vi "GV-progress.vi"() -> (6 "37x37":picture)   [LabVIEW 2020, in "Gviewer.lvclass"]
doc: "Andre Koelewijn, April 2019\n\nThis progress indicator shows loop activity and indicates loop time in msec or seconds.\nExtreme fast loops will increase indicator speed.\nAverage speed loops will show identical indicator speed.\nExtreme slow loops will show by low speed update rate."
uses:
  Gviewer.lvclass
  <vilib>/ptbypt/NI_PtbyPt.lvlib
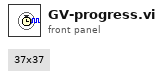
[diagram p1: front panel]
types:
  T1 = cluster{"horizontal":enum16{"left", "center", "right"}, "vertical":enum16{"top", "center", "bottom"}}
  T2 = cluster{"Width":u16, "Style":enum32{"Solid", "Dash", "Dot", "DashDot", "DashDotDot"}}
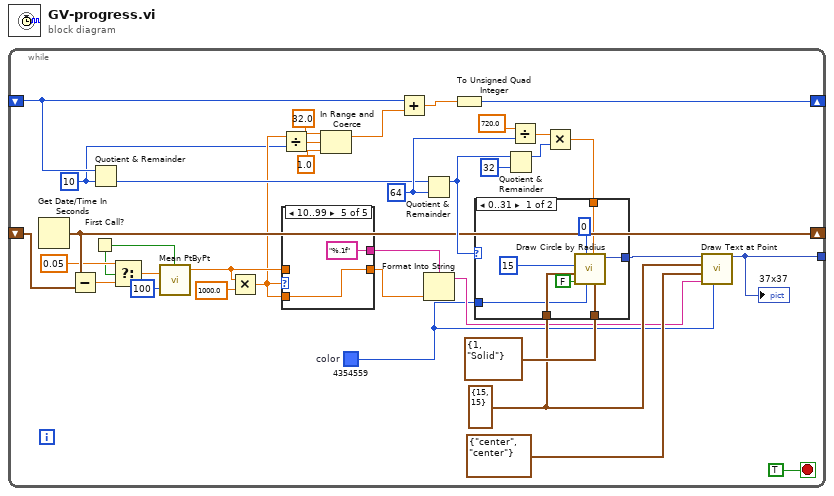
[diagram p0: block diagram]
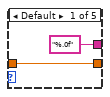
[diagram p2: hidden frame]
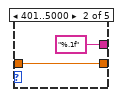
[diagram p3: hidden frame]
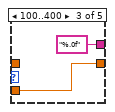
[diagram p4: hidden frame]
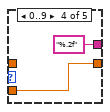
[diagram p5: hidden frame]
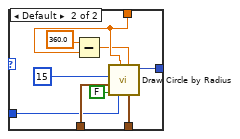
[diagram p6: hidden frame]
diagram:
  n1 = while {
    shift-right: [w23] -> _
    shift-left: _ -> [w27]
    tunnel: [w14] -> _
    shift-right: [w13] -> _
    shift-left: _ -> [w8]
    stop <- TRUE stop-if-true
    w5 = u64 10 ("y")
    w12 = u32 4354559  # color
    w21 = cluster{"horizontal":i16, "vertical":i16} {"horizontal"=15, "vertical"=15} ("pixel center")
    w29 = u64 64 ("y")
    n2 = Get Date/Time In Seconds() -> (seconds since 1Jan1904=w23:timestamp)
    n3 = Subtract(x=w23, y=w27) -> (x-y=w16:dbl)
    n4 = First Call?() -> (First Call?: T/F=w10:bool)
    n5 = Quotient & Remainder(x=w8, y=w5) -> (floor(x/y)=w9:u64)  [unwired: 1 out]
    n6 = Select(t=0.05, s=w10, f=w16) -> (s? t:f=w11:dbl)
    n7 = call <vilib>:"Mean PtByPt.vi"("x"=w11, "sample length"=100, "initialize"=w10) -> ("mean"=w24:dbl)  [unwired: 1 in, 1 out]
    n8 = Multiply(x=w24, y=1000.0) -> (x*y=w6:dbl)
    n9 = Divide(x=w6, y=w5) -> (x/y=w4:dbl)
    n10 = case shown="10..99" w6 {
      tunnel: [w38 w40 w42 w44 w46] -> w19
      tunnel: w6 -> [_ _ w42 w44 w46]
      tunnel: w24 -> [w38 w40 _ _ _]
      tunnel: ["%.0f" ("format string") "%.1f" ("format string") "%.0f" ("format string") "%.2f" ("format string") "%.1f" ("format string")] -> w18
      frame Default {
      }
      frame 401..5000 {
      }
      frame 100..400 {
      }
      frame 0..9 {
      }
      frame 10..99 {
      }
    }
    n11 = In Range and Coerce(upper limit=32.0, x=w4, lower limit=1.0) -> (coerced(x)=w1:dbl)  [unwired: 1 out]
    n12 = Add(x=w8, y=w1) -> (x+y=w7:dbl)
    n13 = Quotient & Remainder(x=w9, y=w29) -> (x-y*floor(x/y)=w28:u64)  [unwired: 1 out]
    n14 = Format Into String(format string=w18, w19) -> (resulting string=w17:string)  [unwired: 2 in, 1 out]
    n15 = To Unsigned Quad Integer(1:w7) -> (0:w13:u64)
    n16 = Quotient & Remainder(x=w28, y=u64 32) -> (x-y*floor(x/y)=w31:u64)  [unwired: 1 out]
    n17 = Divide(x=720.0, y=w29) -> (x/y=w34:dbl)
    n18 = Multiply(x=w34, y=w31) -> (x*y=w30:dbl)
    n19 = case shown="0..31" w28 {
      tunnel: [w54 w63] -> w22
      tunnel: w30 -> [w51 w58]
      tunnel: T2 {"Width"=1, "Style"=enum."Solid"} ("pen") -> [w49 w60]
      tunnel: w21 -> [w48 w56]
      tunnel: w12 -> [w47 w55]
      frame 0..31 {
        n20 = call <vilib>:"Draw Circle by Radius.vi"("pen"=w49, "arc size(360)"=w51, "color(black)"=w47, "start angle(0)"=i16 0, "fill?(F)"=FALSE, "pixel center"=w48, "radius"=i16 15) -> ("new picture"=w54:picture)  [unwired: 4 in]
      }
      frame Default {
        n21 = Subtract(x=360.0 ("start angle(0)"), y=w58) -> (x-y=w57:dbl)
        n22 = call <vilib>:"Draw Circle by Radius.vi"("pen"=w60, "arc size(360)"=w57, "color(black)"=w55, "start angle(0)"=w58, "fill?(F)"=FALSE, "pixel center"=w56, "radius"=i16 15) -> ("new picture"=w63:picture)  [unwired: 4 in]
      }
    }
    n23 = call <vilib>:"Draw Text at Point.vi"("text color(black)"=w12, "text"=w17, "alignment(left, top)"=T1 {"horizontal"=enum."center", "vertical"=enum."center"}, "origin"=w21, "picture"=w22) -> ("new picture"=w14:picture)  [unwired: 5 in, 1 out]
    "37x37" <- w14
  }
